vi "SXM.vi"(1 "Path":path, 2 "Delete":bool, 3 "error in":errorcluster) -> (10 "error out":errorcluster)   [LabVIEW 2014]
uses:
  <userlib>/Nanonis Prog Interface V5/Nanonis Prog Interface.lvlib
panel:
  in  "Scan direction":bool=TRUE
  in  "string":string="A"
  in  "Filename control":cluster{"Path":path, "Basename":string}={"Path"=path "C:/", "Basename"="unnamed"}
  in  "Read channel":i8 min=-1
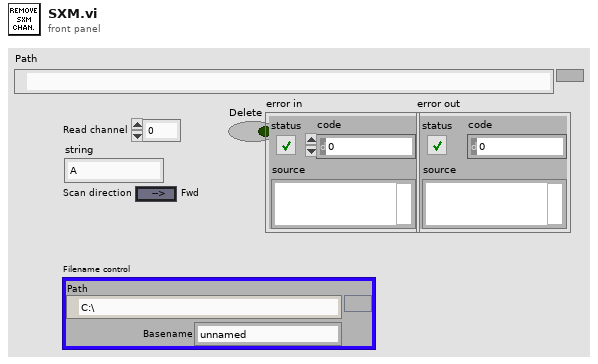
[diagram p1: front panel]
types:
  T1 = cluster{"Name":string, "Calibration":sgl, "Offset":sgl, "Channel index":i32}[]
  T2 = cluster{"center X":sgl, "center Y":sgl, "angle":sgl, "width":sgl, "height":sgl, "# pixels":i32, "# lines":i32}
  T3 = cluster{"up/down":bool, "time/line":sgl, "starttime":timestamp, "endtime":timestamp}
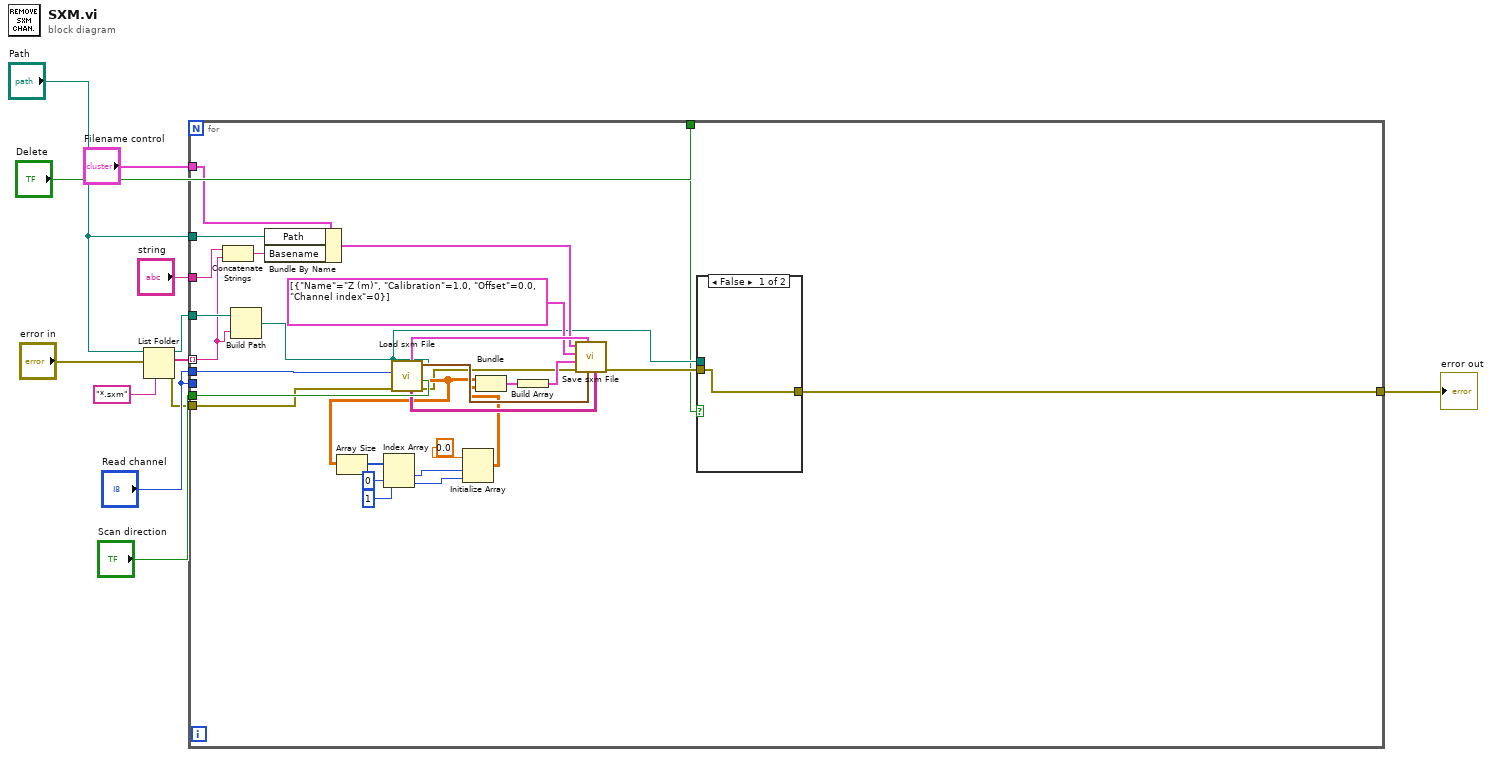
[diagram p0: block diagram]
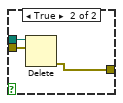
[diagram p2: hidden frame]
diagram:
  n1 = List Folder(path="Path", pattern="*.sxm", error in="error in") -> (path out=w5:path, filenames=w11:string[], error out=w2:errorcluster)  [unwired: 1 in, 1 out]
  n2 = for {
    tunnel: w11 -> [w27] mode=indexing
    tunnel: "Read channel" -> [w41]
    tunnel: "Filename control" -> [w40]
    tunnel: "Path" -> [w39]
    tunnel: "string" -> [w37]
    tunnel: "Scan direction" -> [w36]
    tunnel: "Read channel" -> [_]
    tunnel: w5 -> [w28]
    tunnel: "Delete" -> [w16]
    tunnel: w2 -> [w15]
    tunnel: [w13] -> w1
    n3 = Concatenate Strings(w37, w27) -> (w38:string)
    n4 = Build Path(base path=w28, name or relative path=w27) -> (appended path=w26:path)
    n5 = Bundle By Name(cluster=w40, "Path"=w39, "Basename"=w38) -> (w29:cluster{"Path":path, "Basename":string})
    n6 = call <userlib>:"Load sxm File.vi"("error in"=w15, "Scan direction"=w36, "Read channel"=w41, "Scan data file"=w26) -> ("error out"=w14:errorcluster, "Data"=w23:sgl[][], "Scanfield"=w32:T2, "Parameters"=w34:string[][], "Scan param"=w35:T3)  [unwired: 2 in, 1 out]
    n7 = Array Size(array=w23) -> (size(s)=w22:i32[])
    n8 = Index Array(array=w22, index #1=0 ("index"), index #2=1 ("index")) -> (element #1=w19:i32, element #2=w18:i32)
    n9 = Initialize Array(0.0 ("element"), w19, w18) -> (w17:dbl[][])
    n10 = Bundle("Data"=w23, w17) -> (w31:cluster{"Data":sgl[][], dbl[][]})  [unwired: 1 in]
    n11 = Build Array(w31) -> (w30:cluster{"Data":sgl[][], dbl[][]}[])
    n12 = call <userlib>:"Save sxm File.vi"("Parameters"=w34, "Scanfield"=w32, "Scan param"=w35, "error in (no error)"=w14, "Channels data"=w30, "Channels config"=T1 [{"Name"="Z (m)", "Calibration"=1.0, "Offset"=0.0, "Channel index"=0}], "Filename control"=w29) -> ("error out"=w25:errorcluster)  [unwired: 2 in, 2 out]
    n13 = case shown="False" w16 {
      tunnel: w26 -> [_ w45]
      tunnel: w25 -> [w42 w44]
      tunnel: [w42 w43] -> w13
      frame False {
      }
      frame True {
        n14 = Delete(path (use dialog)=w45, error in=w44) -> (error out=w43:errorcluster)  [unwired: 3 in, 2 out]
      }
    }
  }
  "error out" <- w1
